vi "add_numbers.vi"(8 "error in":errorcluster, 11 "JSON Tree In (JSON Object)":variant) -> (0 "error out":errorcluster, 2 "result":variant, 3 "JSON Tree Out Passthrough":variant)   [LabVIEW 2010]
uses:
  src/i3-json-1.0.0-10/JSON Parsing/Get Object Parameter Files/Get Object Parameter - Object.vi
  src/i3-json-1.0.0-10/JSON Parsing/Get Object Parameter Files/Get Object Parameter - Numeric.vi
  src/i3-json-1.0.0-10/JSON Generation/Create Value Files/Create Value - Numeric.vi
  src/i3-json-1.0.0-10/i3-json.lvlib
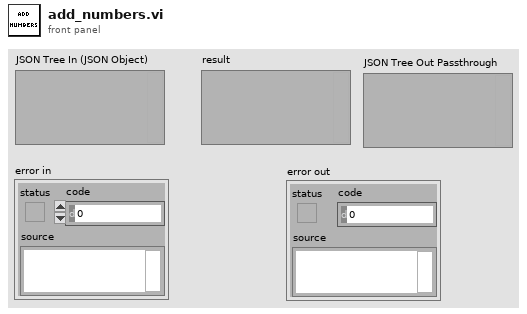
[diagram p1: front panel]
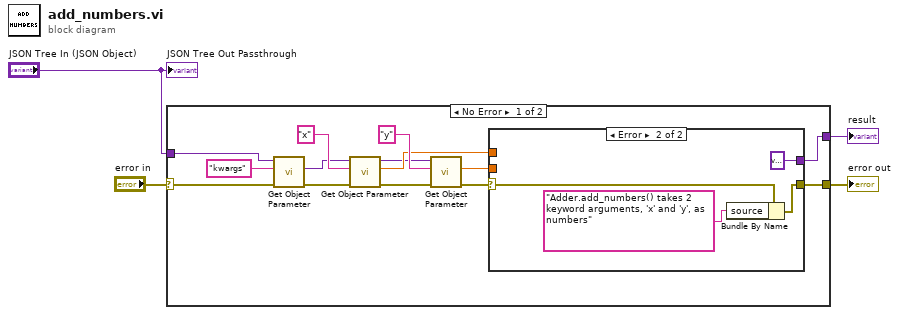
[diagram p0: block diagram]
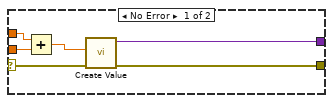
[diagram p2: hidden frame]
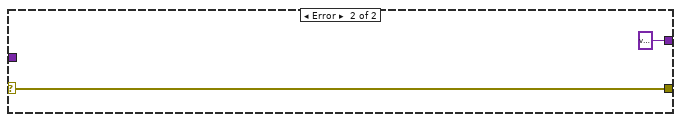
[diagram p3: hidden frame]
diagram:
  n1 = case shown="No Error" "error in" {
    selector: "error in" -> [w15 w30]
    tunnel: "JSON Tree In (JSON Object)" -> [w16 _]
    tunnel: [w13 variant ("JSON Tree In (JSON Object)")] -> w4
    tunnel: [w12 w30] -> w2
    frame No Error {
      n2 = call-poly "Get Object Parameter.vi"("error in (no error)"=w15, "Parameter Name"="kwargs", "JSON Tree In (JSON Object)"=w16) -> ("error out"=w8:errorcluster, "JSON Object"=w9:variant)  [unwired: 5 in, 2 out]
      n3 = call-poly "Get Object Parameter.vi"("error in (no error)"=w8, "Parameter Name"="x", "JSON Tree In (JSON Object)"=w9) -> ("error out"=w7:errorcluster, "Double Value"=w10:dbl, "JSON Tree Out Passthrough"=w6:variant)  [unwired: 5 in, 1 out]
      n4 = call-poly "Get Object Parameter.vi"("error in (no error)"=w7, "Parameter Name"="y", "JSON Tree In (JSON Object)"=w6) -> ("error out"=w5:errorcluster, "Double Value"=w14:dbl)  [unwired: 5 in, 2 out]
      n5 = case shown="Error" w5 {
        selector: w5 -> [w19 w27]
        tunnel: w14 -> [w24 _]
        tunnel: [w22 variant ("JSON Tree")] -> w13
        tunnel: [w21 w26] -> w12
        tunnel: w10 -> [w20 _]
        frame No Error {
          n6 = Add(x=w20, y=w24) -> (x+y=w23:dbl)
          n7 = call-poly "Create Value.vi"("error in (no error)"=w19, "Numeric"=w23) -> ("error out"=w21:errorcluster, "JSON Tree"=w22:variant)  [unwired: 8 in]
        }
        frame Error {
          n8 = Bundle By Name(cluster=w27, "source"="Adder.add_numbers() takes 2 keyword arguments, 'x' and 'y', as numbers") -> (w26:errorcluster)
        }
      }
    }
    frame Error {
    }
  }
  "result" <- w4
  "error out" <- w2
  "JSON Tree Out Passthrough" <- "JSON Tree In (JSON Object)"
